vi "String to Snake Case.vi"(11 "String":string) -> (3 "Snake Case String":string)   [LabVIEW 2020, in "Omega Platinum Series Plugin.lvlib" / "Logging.lvlib"]
uses:
  Logging.lvlib
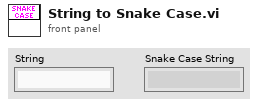
[diagram p1: front panel]
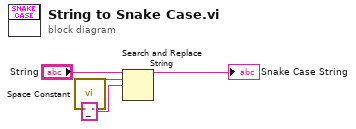
[diagram p0: block diagram]
diagram:
  n1 = call <vilib>:"Space Constant.vi"() -> ("String"=w3:string)
  n2 = Search and Replace String(input string="String", search string=w3, replace string="_" ("replace string (\"\")")) -> (result string=→"Snake Case String":string)  [unwired: 5 in, 3 out]
